vi "Callback Change Channel Name.vi"(6 "Variant":variant, 8 "error in (no error)":errorcluster, 9 "old values":string[][](array[string]), 10 "object ref in":T1, 11 "Cluster":T2) -> (0 "error out":errorcluster)   [LabVIEW 2014, in "tag bus configurable plugin editor node.lvclass"]
uses:
  tag bus configurable plugin editor node.lvclass
  Table Manager/Cell Change.ctl
  Table Manager/object ref.ctl
  Configuration Editor/Classes/Engine Parent/Engine Parent Editor Node.lvclass
  Configuration Editor/Classes/Module editor node/module editor node.lvclass
  module/configuration/tag bus configurable plugin module configuration.lvclass
  module/configuration/tag bus configurable plugin module configuration.lvclass/tag bus configurable plugin module configuration.ctl
  <vilib>/NI/Tag Bus/tag/tag descriptor.lvclass/tag descriptor.ctl
  module/configuration/Find Duplicate.vi
  module/configuration/Get Line Name.vi
  <vilib>/Utility/error.llb/Error Cluster From Error Code.vi
  <vilib>/NI/Tag Bus Module Framework/channel/TBM channel.lvclass
  <vilib>/NI/Tag Bus/tag/tag descriptor.lvclass
  Table Manager.lvlib
  Table Manager/Table Manager.lvclass
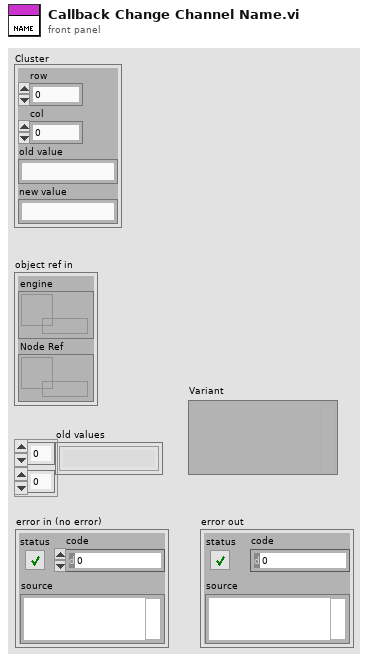
[diagram p1: front panel]
types:
  T1 = typedef "Table Manager.lvlib/Table Manager.lvclass/object ref.ctl" = cluster{"engine":refnum<data-value>, "Node Ref":refnum<data-value>}
  T2 = typedef "Table Manager.lvlib/Cell Change.ctl" = cluster{"row":i32, "col":i32, "old value":string, "new value":string}
  T3 = typedef "tag bus configurable plugin module configuration.lvclass/Line.ctl" = cluster{"channel":refnum<class "TBM channel.lvclass">}
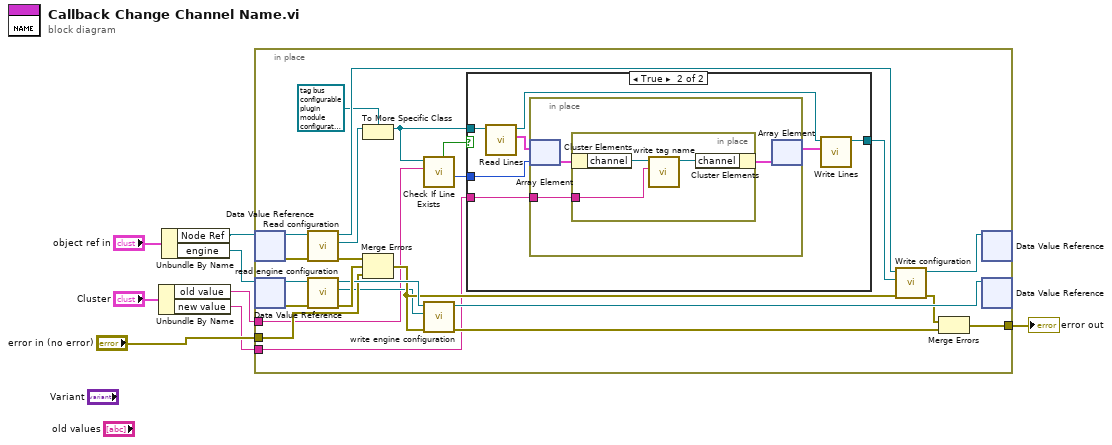
[diagram p0: block diagram]
diagram:
  n1 = Unbundle By Name("Cluster") -> ("old value"=w2:string, "new value"=w1:string)
  n2 = Unbundle By Name("object ref in") -> ("Node Ref"=w5:refnum<data-value>, "engine"=w4:refnum<data-value>)
  n3 = in-place {
    in-place-border: [w24] -> w8
    in-place-border: "error in (no error)" -> [w18]
    in-place-border: w2 -> [w15]
    in-place-border: w1 -> [w11]
    n4 = in-place-dvr #1(w5) -> (w9:refnum<class "module editor node.lvclass">, w23:errorcluster)
    n5 = in-place-dvr #2(w4) -> (w31:refnum<class "Engine Parent Editor Node.lvclass">, w32:errorcluster)
    n6 = call-dynamic "Read configuration.vi"("error in"=w23, "NISE_CEF_serializable node in"=w9) -> ("error out"=w22:errorcluster, "configuration"=w20:refnum<class "NISE_CEF_serializable configuration.lvclass">, "NISE_CEF_serializable node out"=w21:refnum<class "module editor node.lvclass">)  [unwired: 7 in]
    n7 = call "read engine configuration.vi"("error in"=w32, "Engine Parent Editor Node in"=w31) -> ("error out"=w28:errorcluster, "engine configuration"=w17:refnum<class "engine configuration.lvclass">, "Engine Parent Editor Node out"=w27:refnum<class "Engine Parent Editor Node.lvclass">)  [unwired: 7 in]
    n8 = To More Specific Class(target class=refnum<class "tag bus configurable plugin module configuration.lvclass"> refnum ("tag bus configurable plugin module configuration"), reference=w20) -> (specific class reference=w13:refnum<class "tag bus configurable plugin module configuration.lvclass">)  [unwired: 1 in, 1 out]
    n9 = Merge Errors(w22, w28, w18) -> (w19:errorcluster)
    n10 = call-dynamic "Check If Line Exists.vi"("name to locate"=w15, "tag bus configurable plugin module configuration in"=w13) -> ("index"=w12:i32, "found?"=w10:bool)  [unwired: 5 in, 3 out]
    n11 = call "write engine configuration.vi"("error in"=w19, "engine configuration"=w17, "Engine Parent Editor Node in"=w27) -> ("error out"=w26:errorcluster, "Engine Parent Editor Node out"=w30:refnum<class "Engine Parent Editor Node.lvclass">)  [unwired: 7 in]
    n12 = case shown="True" w10 {
      tunnel: [w33 w40] -> w14
      tunnel: w13 -> [w33 w38]
      tunnel: w12 -> [_ w35]
      tunnel: w11 -> [_ w34]
      frame False {
      }
      frame True {
        n13 = call "Read Lines.vi"("tag bus configurable plugin module configuration in"=w38) -> ("Lines"=w37:T3[], "tag bus configurable plugin module configuration out"=w39:refnum<class "tag bus configurable plugin module configuration.lvclass">)  [unwired: 8 in, 1 out]
        n14 = in-place {
          in-place-border: w34 -> [w41]
          n15 = in-place-array #3(w37, w35) -> (w43:T3)
          n16 = in-place {
            in-place-border: w41 -> [w44]
            n17 = in-place-cluster #4(w43) -> ("channel"=w46:refnum<class "TBM channel.lvclass">)
            n18 = call <vilib>:"write tag name.vi"("name"=w44, "system tag in"=w46) -> ("system tag out"=w45:refnum<class "TBM channel.lvclass">)  [unwired: 8 in, 1 out]
            n19 = in-place-cluster #4("channel"=w45) -> (w42:T3)
          }
          n20 = in-place-array #3(w42) -> (w36:T3[])  [unwired: 1 out]
        }
        n21 = call "Write Lines.vi"("Lines"=w36, "tag bus configurable plugin module configuration in"=w39) -> ("tag bus configurable plugin module configuration out"=w40:refnum<class "tag bus configurable plugin module configuration.lvclass">)  [unwired: 8 in, 1 out]
      }
    }
    n22 = call-dynamic "Write configuration.vi"("error in"=w19, "configuration"=w14, "NISE_CEF_serializable node in"=w21) -> ("error out"=w25:errorcluster, "NISE_CEF_serializable node out"=w29:refnum<class "module editor node.lvclass">)  [unwired: 7 in]
    n23 = Merge Errors(w25, w26) -> (w24:errorcluster)
    n24 = in-place-dvr #1(w29) -> ()  [unwired: 2 out]
    n25 = in-place-dvr #2(w30) -> ()  [unwired: 2 out]
  }
  "error out" <- w8
